vi "INIT_HP.vi"(4 "Averaging Number (8:256)":u32(ring) items=["1", "2", "4", "8", "16", "32", "64", "128", "256"], 6 "Integration Time":u32(ring)=2 items=["Short", "Medium", "Long"], 7 "Osc_Level [V]":dbl=0.02, 8 "BIAS [V]":dbl=15.0 format="%#_13g", 9 "Set":u32(ring)=7 caption="Selection A-B:" items=["| Z | -Ttheta ", "R - X", "Ls-Rs", "Ls-Q", "Cs-Rs", "Cs-Q", "Cs-D", "|Y|-Theta", "G-B", "Lp-G", "Lp-Q", "Cp-G", "Cp-Q", "Cp-D", "|Z|-Ls", "|Z|-Cs", "|Z|-Lp", "|Z|-Cp", "Lp-Rp", "Cp-Rp"], 10 "Reset Device (T:Reset Device)":bool, 11 "Type":u32(ring) caption="Measurement type" items=["Impedance ", "Gain - Phase", "Impedance With Probe"]) -> (0 "error out":errorcluster, 3 "VISA Refnum out":refnum<visa-resource-name>)   [LabVIEW 2017]
uses:
  Agilent 4194/Agilent 4194.lvlib
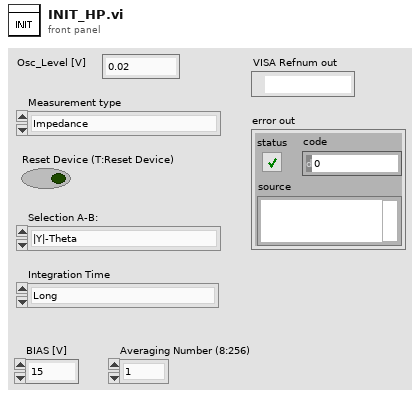
[diagram p1: front panel]
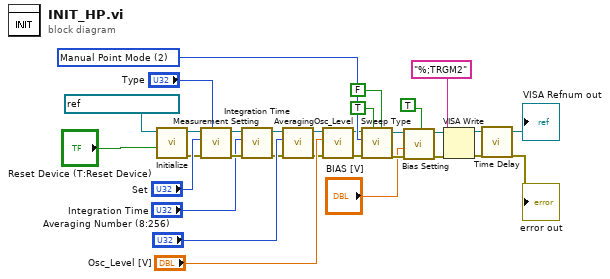
[diagram p0: block diagram]
diagram:
  w17 = u32 2 items=["Repeat", "Single", "Manual Point Mode"] ("Sweep Mode (0:Repeat)")
  n1 = call "Initialize.vi"("Reset Device (T:Reset Device)"="Reset Device (T:Reset Device)", "VISA resource name"=refnum<visa-resource-name> "GPIB0::17::INSTR") -> ("error out"=w3:errorcluster, "VISA resource name out"=w2:refnum<visa-resource-name>)  [unwired: 8 in]
  n2 = call "Measurement Setting.vi"("Measurement Type (0:Impedance)"="Type", "error in (no error)"=w3, "Impedance (0:| Z | - Theta )"="Set", "VISA resource name"=w2) -> ("error out"=w30:errorcluster, "VISA resource name out"=w29:refnum<visa-resource-name>)  [unwired: 6 in]
  n3 = call "Integration Time.vi"("error in (no error)"=w30, "Integration Time (0:Short)"="Integration Time", "VISA resource name"=w29) -> ("error out"=w6:errorcluster, "VISA resource name out"=w5:refnum<visa-resource-name>)  [unwired: 7 in]
  n4 = call "Averaging.vi"("error in (no error)"=w6, "Averaging Number (8:256)"="Averaging Number (8:256)", "VISA resource name"=w5) -> ("error out"=w9:errorcluster, "VISA resource name out"=w8:refnum<visa-resource-name>)  [unwired: 7 in]
  n5 = call "Osc_Level.vi"("error in (no error)"=w9, "Osc_Level [V]"="Osc_Level [V]", "VISA resource name"=w8) -> ("error out"=w14:errorcluster, "VISA resource name out"=w13:refnum<visa-resource-name>)  [unwired: 7 in]
  n6 = call "Sweep Type.vi"("Sweep Type (F:Linear)"=FALSE, "Sweep Direction (F:Down)"=TRUE, "error in (no error)"=w14, "Sweep Mode (0:Repeat)"=w17, "VISA resource name"=w13) -> ("error out"=w23:errorcluster, "VISA resource name out"=w22:refnum<visa-resource-name>)  [unwired: 5 in]
  n7 = call "Bias Setting.vi"("error in (no error)"=w23, "DC Bias Value (0.0 V)"="BIAS [V]", "DC Bias (F:Off)"=TRUE, "VISA resource name"=w22) -> ("error out"=w20:errorcluster, "VISA resource name out"=w19:refnum<visa-resource-name>)  [unwired: 6 in]
  n8 = VISA Write(VISA resource name=w19, write buffer="%;TRGM2", error in (no error)=w20) -> (VISA resource name out=→"VISA Refnum out":refnum<visa-resource-name>, error out=w18:errorcluster)  [unwired: 1 out]
  n9 = call "Time Delay"("error in (no error)"=w18) -> ("error out"=→"error out":errorcluster)  [unwired: 10 in]
